vi "CreateFileHandler.vi"(4 "Delay":bool, 5 "Mode":string, 6 "Errors":string, 7 "FIlePath":path, 8 "error in (no error)":errorcluster, 9 "Encoding":string, 10 "Name":string, 11 "Logger in":refnum<class "Logger.lvclass">) -> (0 "error out":errorcluster, 2 "FileHandler":refnum<class "FileHandler.lvclass">, 3 "Logger out":refnum<class "Logger.lvclass">)   [LabVIEW 2022 SP3, in "Logger.lvlib" / "Logger.lvclass"]
uses:
  Logger.lvclass
  C:/Users/jakub/repos/gh/sw4sys/lv-logger/Logger/Source/LoggingWrapper/LoggingWrapper.lvclass
  C:/Users/jakub/repos/gh/sw4sys/lv-logger/PythonWrapper/Source/PythonSession/PythonSession.lvclass
  C:/Users/jakub/repos/gh/sw4sys/lv-logger/PythonWrapper/Source/PythonWrapper/PythonWrapper.lvclass
  FileHandler/FileHandler.lvclass
  C:/Users/jakub/repos/gh/sw4sys/lv-logger/Logger/Source/Handler/Handler.lvclass
  LoggingWrapper/LoggingWrapper.lvclass/LoggingWrapper.ctl
  PythonWrapper/Source/PythonSession/PythonSession.lvclass/PythonSession.ctl
  PythonWrapper/Source/PythonWrapper/PythonWrapper.lvclass/PythonWrapper.ctl
  Handler/Handler.lvclass/Handler.ctl
  LoggingWrapper/Read FunctionSetFormatter.vi
  LoggingWrapper/Read FunctionSetHandlerLevel.vi
  PythonWrapper/Source/PythonSession/Read PythonSession.vi
  PythonWrapper/Source/PythonWrapper/Read ModulePath.vi
  Handler/Write FunctionSetFormatter.vi
  Handler/Write FunctionSetHandlerLevel.vi
  Handler/Write PythonSession.vi
  Handler/Write ModulePath.vi
  Handler/Write Name.vi
  Logger.lvclass/Logger.ctl
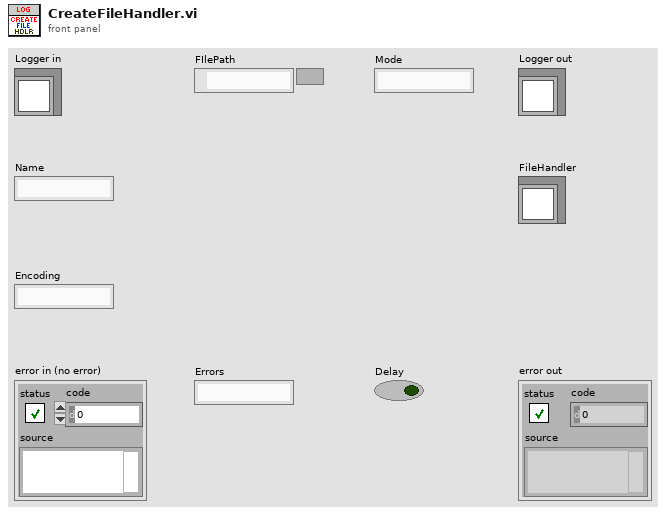
[diagram p1: front panel]
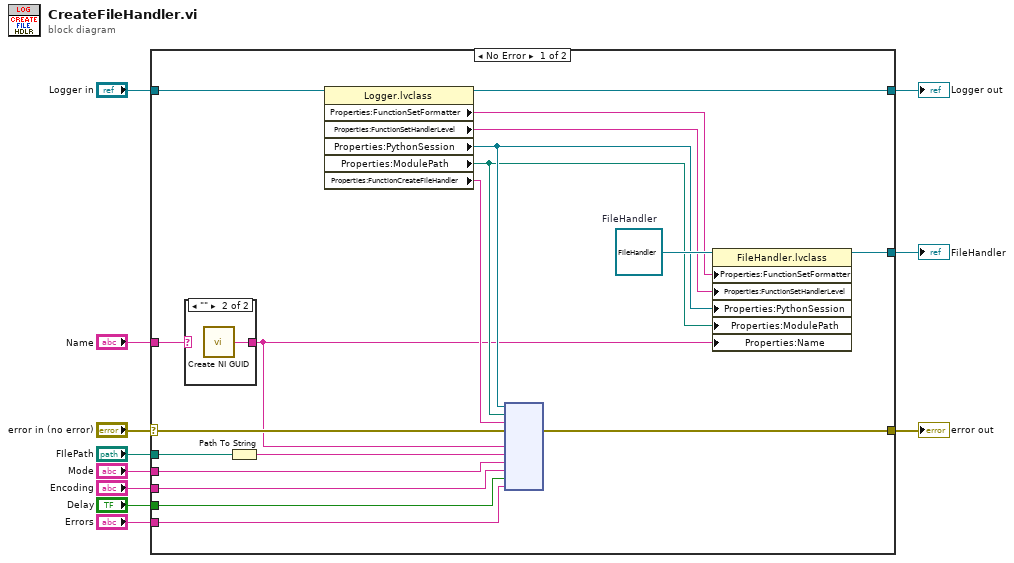
[diagram p0: block diagram]
diagram:
  n1 = case shown="No Error" "error in (no error)" {
    selector: "error in (no error)" -> [w28 w34]
    tunnel: [w25 w34] -> w8
    tunnel: [w29 w33] -> w10
    tunnel: "Logger in" -> [w30 w33]
    tunnel: "FIlePath" -> [w26 _]
    tunnel: "Mode" -> [w14 _]
    tunnel: "Encoding" -> [w15 _]
    tunnel: "Delay" -> [w16 _]
    tunnel: "Errors" -> [w17 _]
    tunnel: [w18 _] -> w2
    tunnel: "Name" -> [w19 _]
    frame No Error {
      w24 = refnum<class "FileHandler.lvclass"> refnum  # FileHandler
      n2 = case shown="\"\"" w19 {
        selector: w19 -> [w31 _]
        tunnel: [w31 w32] -> w12
        frame Default {
        }
        frame "" {
          n3 = call <vilib>:"Create NI GUID.vi"() -> ("NI GUID"=w32:string)
        }
      }
      n4 = Path To String(path=w26) -> (string=w13:string)
      n5 = property class="Logger.lvclass"(reference=w30) -> (reference out=w29:refnum<class "Logger.lvclass">, "Properties:FunctionSetFormatter"=w23:string, "Properties:FunctionSetHandlerLevel"=w22:string, "Properties:PythonSession"=w21:refnum<k35>, "Properties:ModulePath"=w20:path, "Properties:FunctionCreateFileHandler"=w27:string)  [unwired: 1 in, 1 out]
      n6 = node(w21, w20, w27, w28, w12, w13, w14, w15, w16, w17) -> (w25:errorcluster)  [unwired: 8 in, 3 out]
      n7 = property class="FileHandler.lvclass"(reference=w24, "Properties:FunctionSetFormatter"=w23, "Properties:FunctionSetHandlerLevel"=w22, "Properties:PythonSession"=w21, "Properties:ModulePath"=w20, "Properties:Name"=w12) -> (reference out=w18:refnum<class "FileHandler.lvclass">)  [unwired: 1 in, 1 out]
    }
    frame Error {
    }
  }
  "error out" <- w8
  "Logger out" <- w10
  "FileHandler" <- w2
